vi "GetRunningServerErrors.vi"(8 "error release notification":errorcluster, 9 "error release queue":errorcluster, 10 "error close reference":errorcluster, 11 "server":T1={"vi name"="", "queue"=refnum, "ROS"={"topic port"=0, "Node"="", "topic"="", "type"="", "node port"=0, "error "={"status"=FALSE, "code"=0, "source"=""}, "Direction"=enum."Node", "Update (ms)"=1, "FIFO size"=1}, "notifier"=refnum, "FIFO"=refnum, "This VI"=refnum, "MyState"=enum."No Connection"}) -> ()   [LabVIEW 2012]
doc: "Outputs errors from running servers"
uses:
  SubVIs/_ROSDirection.ctl
  SubVIs/_ROSControl.ctl
  Console/Servers/ServerSubs/ServoInfo.ctl
  Console/Servers/ServerSubs/MyState.ctl
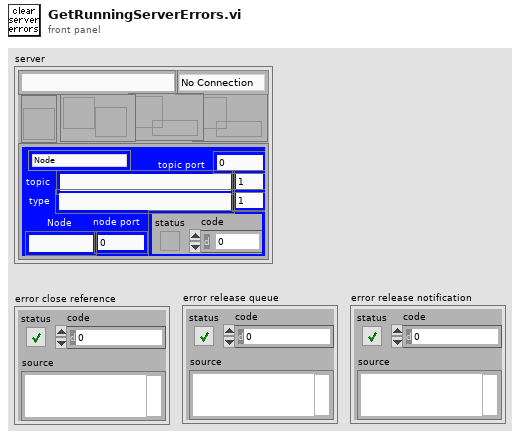
[diagram p1: front panel]
types:
  T1 = typedef "ServoInfo.ctl" = cluster{"vi name":string, "queue":refnum<queue>, "ROS":T2, "notifier":refnum<notifier>, "FIFO":refnum<queue>, "This VI":refnum<vi>, "MyState":T4}
  T2 = typedef "_ROSControl.ctl" = cluster{"topic port":u16, "Node":string, "topic":string, "type":string, "node port":u16, "error ":errorcluster, "Direction":T3, "Update (ms)":u16, "FIFO size":u16}
  T3 = typedef "_ROSDirection.ctl" = enum16{"Node", "Publisher", "Subscriber", "ServiceClient", "ServiceProvider"}
  T4 = typedef "MyState.ctl" = enum16{"No Connection", "Registered", "Connected", "Close"}
  T5 = enum16{"open", "replace", "create", "open or create", "replace or create", "replace or create with confirmation"}
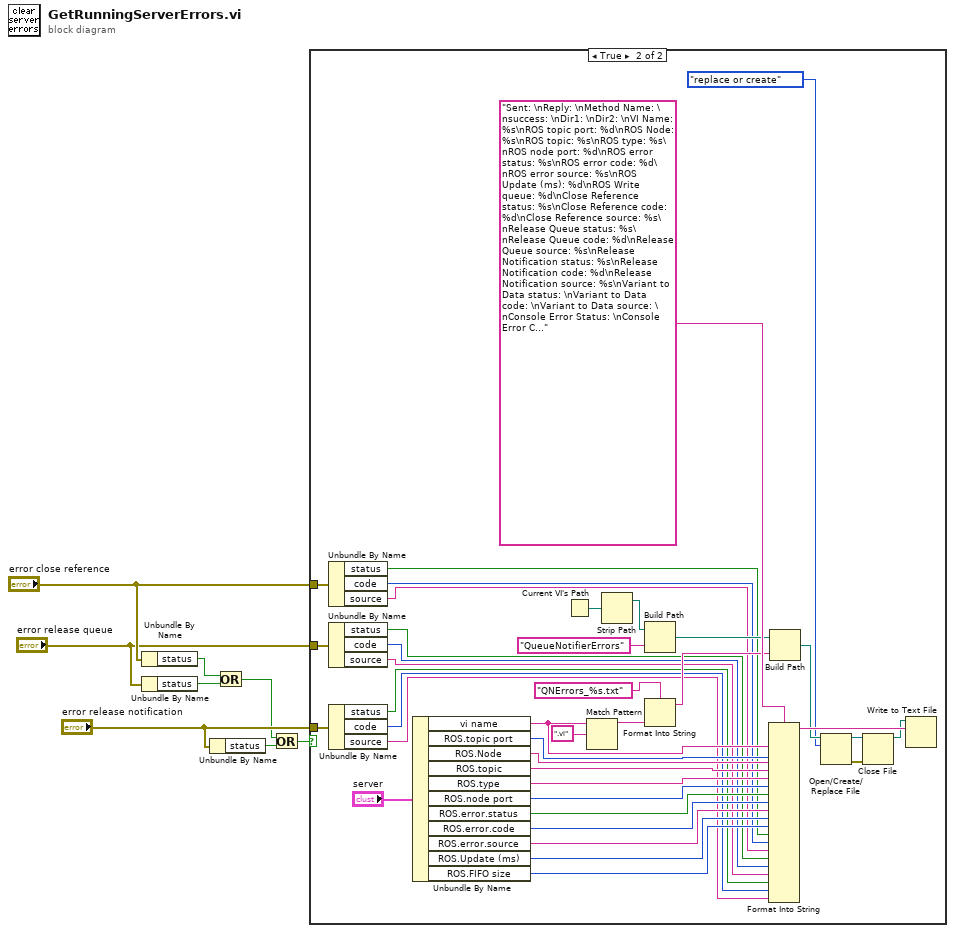
[diagram p0: block diagram]
diagram:
  n1 = Unbundle By Name("error close reference") -> ("status"=w5:bool)
  n2 = Unbundle By Name("error release queue") -> ("status"=w4:bool)
  n3 = Unbundle By Name("error release notification") -> ("status"=w2:bool)
  n4 = Or(x=w5, y=w4) -> (x .or. y?=w3:bool)
  n5 = Or(x=w3, y=w2) -> (x .or. y?=w1:bool)
  n6 = case shown="True" w1 {
    tunnel: "error close reference" -> [_ w20]
    tunnel: "error release queue" -> [_ w19]
    tunnel: "error release notification" -> [_ w18]
    frame False {
    }
    frame True {
      n7 = Unbundle By Name(w20) -> ("status"=w17:bool, "code"=w16:i32, "source"=w15:string)
      n8 = Unbundle By Name(w19) -> ("status"=w14:bool, "code"=w13:i32, "source"=w12:string)
      n9 = Unbundle By Name(w18) -> ("status"=w11:bool, "code"=w10:i32, "source"=w9:string)
      n10 = Unbundle By Name("server") -> ("vi name"=w31:string, "ROS.topic port"=w30:u16, "ROS.Node"=w29:string, "ROS.topic"=w28:string, "ROS.type"=w27:string, "ROS.node port"=w26:u16, "ROS.error.status"=w25:bool, "ROS.error.code"=w24:i32, "ROS.error.source"=w23:string, "ROS.Update (ms)"=w22:u16, "ROS.FIFO size"=w21:u16)
      n11 = Current VI's Path() -> (path=w45:path)
      n12 = Match Pattern(string=w31, regular expression=".vi") -> (before substring=w32:string)  [unwired: 1 in, 3 out]
      n13 = Strip Path(path=w45) -> (stripped path=w44:path)  [unwired: 1 out]
      n14 = Build Path(base path=w44, name or relative path="QueueNotifierErrors") -> (appended path=w42:path)
      n15 = Format Into String(format string="QNErrors_%s.txt", w32) -> (resulting string=w35:string)  [unwired: 2 in, 1 out]
      n16 = Format Into String(format string="Sent: \nReply: \nMethod Name: \nsuccess: \nDir1: \nDir2: \nVI Name: %s\nROS topic port: %d\nROS Node: %s\nROS topic: %s\nROS type: %s\nROS node port: %d\nROS error status: %s\nROS error code: %d\nROS error source: %s\nROS Update (ms): %d\nROS Write queue: %d\nClose Reference status: %s\nClose Reference code: %d\nClose Reference source: %s\nRelease Queue status: %s\nRelease Queue code: %d\nRelease Queue source: %s\nRelease Notification status: %s\nRelease Notification code: %d\nRelease Notification source: %s\nVariant to Data status: \nVariant to Data code: \nVariant to Data source: \nConsole Error Status: \nConsole Error Code: \nConsole Error Source: \nTimestamp: \n====", w31, w30, w29, w28, w27, w26, w25, w24, w23, w22, w21, w17, w16, w15, w14, w13, w12, w11, w10, w9) -> (resulting string=w47:string)  [unwired: 2 in, 1 out]
      n17 = Build Path(base path=w42, name or relative path=w35) -> (appended path=w39:path)
      n18 = Open/Create/Replace File(file path (use dialog)=w39, operation (0:open)=T5."replace or create") -> (refnum out=w40:refnum<file>, error out=w41:errorcluster)  [unwired: 4 in, 1 out]
      n19 = Close File(refnum=w40, error in=w41) -> (path=w37:path)  [unwired: 1 out]
      n20 = Write to Text File(file (use dialog)=w37, text=w47) -> ()  [unwired: 2 in, 3 out]
    }
  }
